vi "Inst.Xeryon-Rotator.Set Speed.vi"(8 "error in (no error)":errorcluster, 10 "Rate (°/min)":dbl, 11 "Inst.Xeryon-Rotator in":refnum<class "Inst.Xeryon-Rotator.lvclass">) -> (0 "error out":errorcluster, 3 "Inst.Xeryon-Rotator out":refnum<class "Inst.Xeryon-Rotator.lvclass">)   [LabVIEW 2019, in "Inst.Xeryon-Rotator.lvclass"]
uses:
  Inst.Xeryon-Rotator.lvclass
  Controller.LV/Controller.LV.lvclass
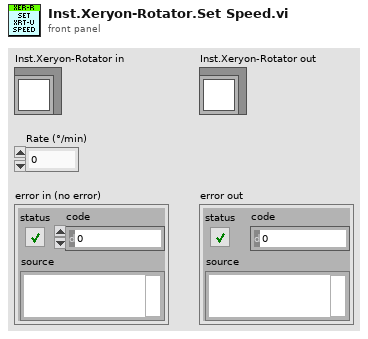
[diagram p1: front panel]
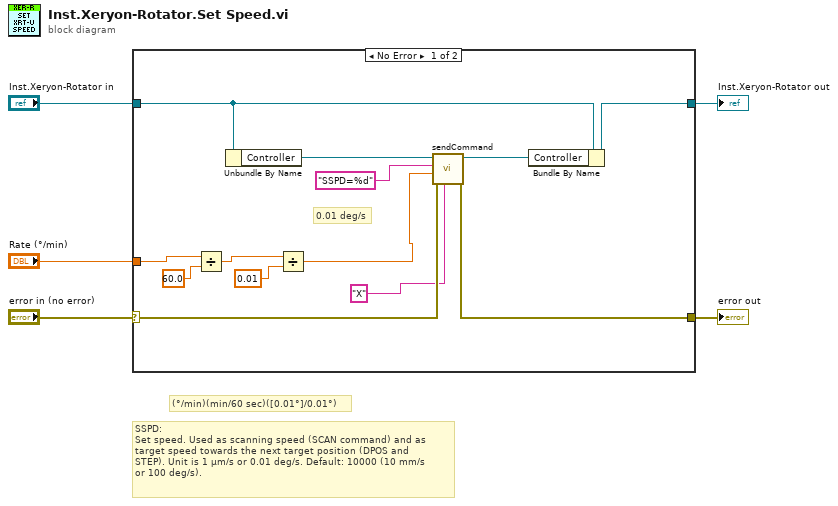
[diagram p0: block diagram]
diagram:
  # "SSPD:\nSet speed. Used as scanning speed (SCAN command) and as\ntarget speed towards the next target position (DPOS and\nSTEP). Unit is 1 µm/s or 0.01 deg/s. Default: 10000 (10 mm/s\nor 100 deg/s)."
  # "(°/min)(min/60 sec)([0.01°]/0.01°)"
  n1 = case shown="No Error" "error in (no error)" {
    selector: "error in (no error)" -> [w9 w20]
    tunnel: [w18 w19] -> w5
    tunnel: "Rate (°/min)" -> [w12 _]
    tunnel: [w11 w20] -> w3
    tunnel: "Inst.Xeryon-Rotator in" -> [w10 w19]
    frame No Error {
      # "0.01 deg/s"
      n2 = Divide(x=w12, y=60.0) -> (x/y=w14:dbl)
      n3 = Unbundle By Name(w10) -> ("Controller"=w16:refnum<class "Controller.LV.lvclass">)
      n4 = Divide(x=w14, y=0.01) -> (x/y=w6:dbl)
      n5 = call-dynamic "sendCommand.vi"("Axis Letter"="X", "error in (no error)"=w9, "Value"=w6, "Command"="SSPD=%d", "Controller in"=w16) -> ("error out"=w11:errorcluster, "Controller out"=w17:refnum<class "Controller.LV.lvclass">)  [unwired: 5 in]
      n6 = Bundle By Name(cluster=w10, "Controller"=w17) -> (w18:refnum<class "Inst.Xeryon-Rotator.lvclass">)
    }
    frame Error {
    }
  }
  "Inst.Xeryon-Rotator out" <- w5
  "error out" <- w3
